vi "BUFMGR_set_released_size.vi"(5 "size in":u64, 11 "error in (no error)":errorcluster) -> (4 "return":u32 format="%.0x", 6 "released buffer":u64, 15 "error out":errorcluster)   [LabVIEW 2016]
uses:
  c/lib/libbuf.so
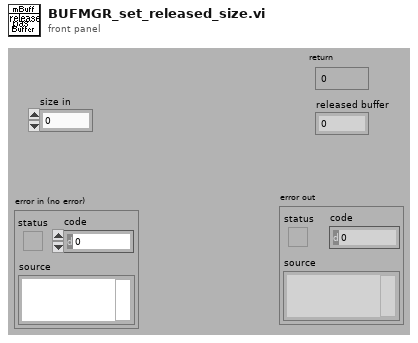
[diagram p1: front panel]
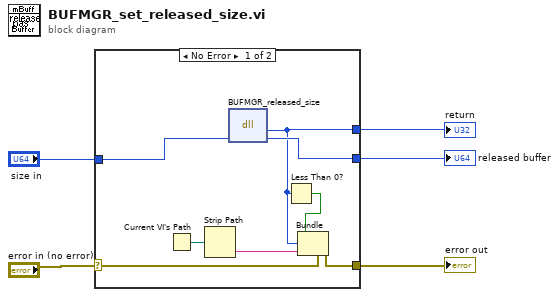
[diagram p0: block diagram]
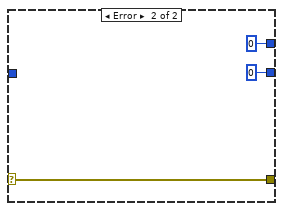
[diagram p2: hidden frame]
diagram:
  n1 = case shown="No Error" "error in (no error)" {
    selector: "error in (no error)" -> [w6 w14]
    tunnel: [w9 u32 0] -> w5
    tunnel: "size in" -> [w13 _]
    tunnel: [w12 0 ("size")] -> w3
    tunnel: [w11 w14] -> w2
    frame No Error {
      n2 = Current VI's Path() -> (path=w8:path)
      n3 = Strip Path(path=w8) -> (name=w7:string)  [unwired: 1 out]
      n4 = dll-call lib="home/simager/panview/PAN/Modules/buffermgr/private/c/lib/libbuf.so" fn="BUFMGR_released_size"("size"=w13) -> ("return type"=w9:u32, "size"=w12:u64)  [unwired: 3 in, 2 out]
      n5 = Less Than 0?(x=w9) -> (x < 0?=w10:bool)
      n6 = Bundle(cluster=w6, "status"=w10, "code"=w9, "source"=w7) -> (w11:errorcluster)
    }
    frame Error {
    }
  }
  "error out" <- w2
  "return" <- w5
  "released buffer" <- w3
